vi "AppConfigTypeToXML.vi"(8 "error in (no error)":errorcluster, 11 "AppPluginsBase in":refnum<class "AppPluginsBase.lvclass">) -> (0 "error out":errorcluster, 2 "ConfigXML out":string, 3 "AppPluginsBase out":refnum<class "AppPluginsBase.lvclass">)   [LabVIEW 2017, in "AppPlugins.lvlib" / "AppPluginsBase.lvclass"]
uses:
  AppPluginsBase.lvclass
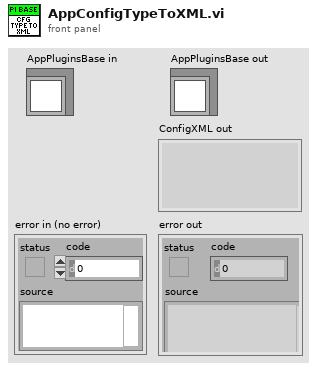
[diagram p1: front panel]
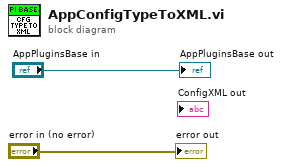
[diagram p0: block diagram]
diagram:
  "error out" <- "error in (no error)"
  "AppPluginsBase out" <- "AppPluginsBase in"
